vi "Raise Conversion Error.vi"(9 "Data Type Attempted":string, 11 "String in Error":string) -> (0 "error out":errorcluster)   [LabVIEW 2023, in "HAF.lvlib"]
doc: "If an attempt to convert a String to a specific Data Type fails, this VI can be used to raise a Framework Error, 205. The message text will look like \"Data Type Conversion Error: cannot convert [String in Error] cannot be converted to [Data Type Attempted]\""
uses:
  HAF.lvlib
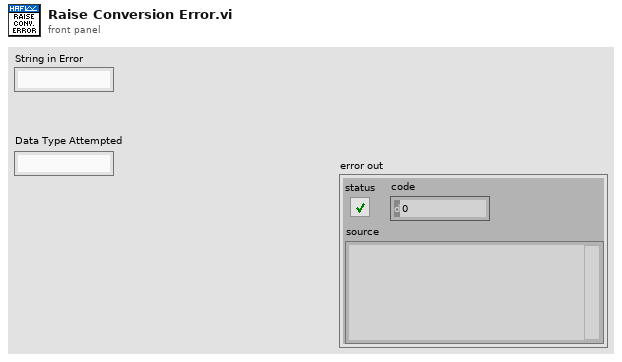
[diagram p1: front panel]
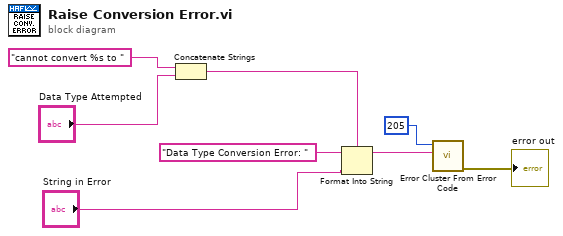
[diagram p0: block diagram]
diagram:
  n1 = Concatenate Strings("cannot convert %s to " ("string"), "Data Type Attempted") -> (w1:string)
  n2 = Format Into String(format string=w1, initial string="Data Type Conversion Error: ", "String in Error") -> (resulting string=w7:string)  [unwired: 1 in, 1 out]
  n3 = call <vilib>:"Error Cluster From Error Code.vi"("error message (\"\")"=w7, "error code (0)"=205) -> ("error out"=→"error out":errorcluster)  [unwired: 7 in]
